vi "[WLC] Calculate Fit.vi"(1 "Temperature (K)":dbl=298.0, 2 "Persistence Length (nm)":dbl, 3 "Contour Length (nm)":dbl) -> (0 "Worm-Like Chain Fit":T1)   [LabVIEW 2013]
uses:
  <vilib>/Analysis/1siggen.llb/Ramp Pattern by Samples.vi
  <vilib>/Analysis/NI_AALBase.lvlib
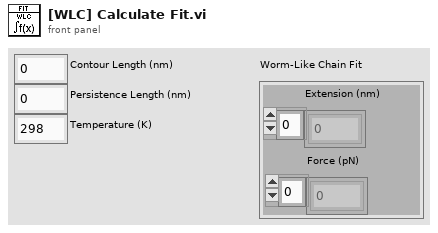
[diagram p1: front panel]
types:
  T1 = cluster{"Extension (nm)":dbl[], "Force (pN)":dbl[]}
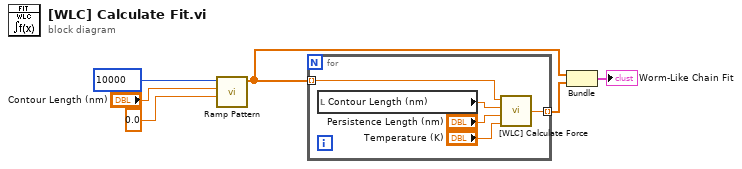
[diagram p0: block diagram]
diagram:
  n1 = call-poly <vilib>:"Ramp Pattern.vi"("start"=0.0, "end"="Contour Length (nm)", "samples"=10000) -> ("Ramp Pattern"=w2:dbl[])  [unwired: 7 in, 1 out]
  n2 = for {
    tunnel: w2 -> [w8] mode=indexing
    tunnel: [w7] -> w3 mode=indexing
    n3 = local read "Contour Length (nm)"() -> (w10:dbl)
    n4 = call "[WLC] Calculate Force.vi"("Temperature (K)"="Temperature (K)", "Persistence Length (nm)"="Persistence Length (nm)", "Contour Length (nm)"=w10, "Extension (nm)"=w8) -> ("Force (pN)"=w7:dbl)
  }
  n5 = Bundle("Ramp Pattern"=w2, w3) -> (→"Worm-Like Chain Fit":cluster{"Ramp Pattern":dbl[], dbl[]})  [unwired: 1 in]
